vi "SetParam.vi"(8 "error in (no error)":errorcluster caption="entrée d'erreur (pas d'erreur)", 10 "scale":T1={"axis"=0, "with_mean"=TRUE, "with_std"=TRUE, "copy"=TRUE}, 11 "scale.lvclass":refnum<class "scale.lvclass">) -> (0 "error out":errorcluster caption="sortie d'erreur", 3 "scale.lvclass":refnum<class "scale.lvclass">)   [LabVIEW 2020, in "scale.lvclass"]
doc: "Set Parameters"
uses:
  scale.lvclass
  scale.lvclass/scale.ctl
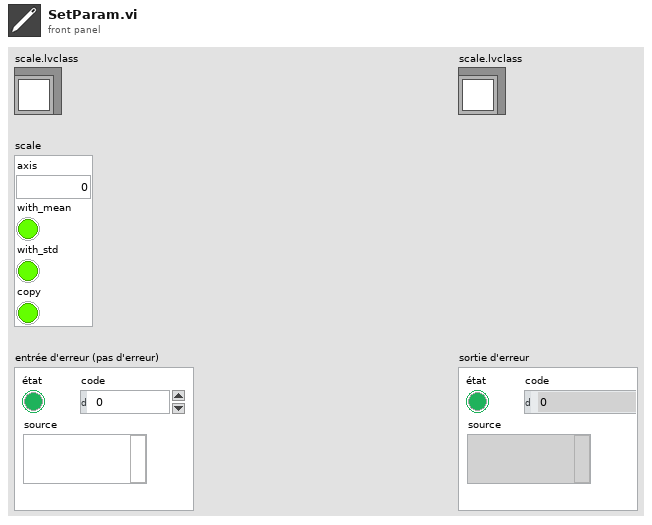
[diagram p1: front panel]
types:
  T1 = cluster{"axis":i32, "with_mean":bool, "with_std":bool, "copy":bool}
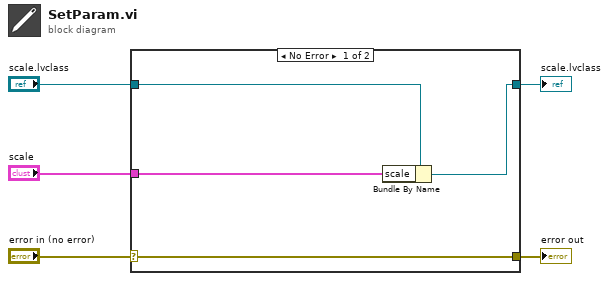
[diagram p0: block diagram]
diagram:
  n1 = case shown="No Error" "error in (no error)" {
    selector: "error in (no error)" -> [w9 w10]
    tunnel: [w9 w10] -> w4
    tunnel: [w7 w11] -> w2
    tunnel: "scale.lvclass" -> [w8 w11]
    tunnel: "scale" -> [w6 _]
    frame No Error {
      n2 = Bundle By Name(cluster=w8, "scale"=w6) -> (w7:refnum<class "scale.lvclass">)
    }
    frame Error {
    }
  }
  "error out" <- w4
  "scale.lvclass" <- w2
